vi "BuildExcelTable.vi"(9 "Names":string[](array[string]), 11 "Value":cluster{dbl, "df":dbl, dbl[]}[](array[cluster])) -> (1 "ColHeaders":string[](array[string]), 3 "Breakdown":string[][](table))   [LabVIEW 2022 SP3]
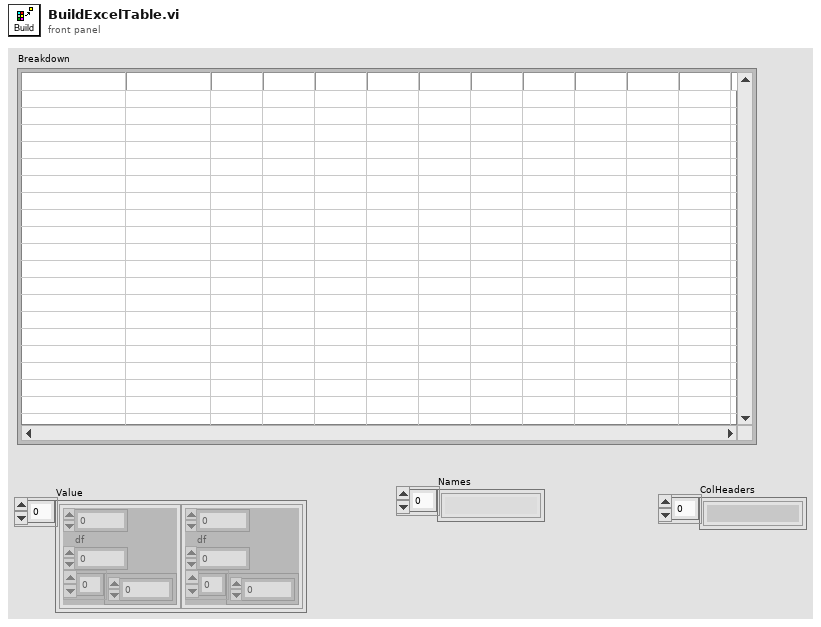
[diagram p1: front panel]
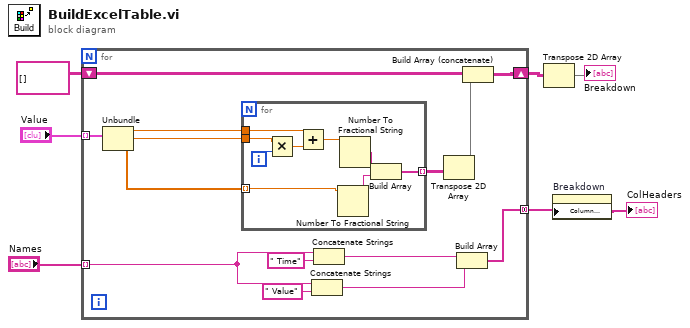
[diagram p0: block diagram]
diagram:
  n1 = for {
    tunnel: "Value" -> [w20] mode=indexing
    shift-right: [w13] -> w2
    shift-left: string[][] [] -> [w12]
    tunnel: [w14] -> w3 mode=concatenating
    tunnel: "Names" -> [w9] mode=indexing
    n2 = Unbundle(w20) -> (w18:dbl, "df"=w19:dbl, w17:dbl[])
    n3 = for {
      tunnel: w19 -> [w28]
      tunnel: w18 -> [w26]
      tunnel: w17 -> [w24] mode=indexing
      tunnel: [w21] -> w16 mode=indexing
      i -> [w29]
      n4 = Multiply(x=w28, y=w29) -> (x*y=w27:dbl)
      n5 = Add(x=w26, y=w27) -> (x+y=w25:dbl)
      n6 = Number To Fractional String(number=w24) -> (F-format string=w23:string)  [unwired: 3 in]
      n7 = Number To Fractional String(number=w25) -> (F-format string=w22:string)  [unwired: 3 in]
      n8 = Build Array(w22, w23) -> (w21:string[])
    }
    n9 = Concatenate Strings(w9, " Value" ("string")) -> (w7:string)
    n10 = Concatenate Strings(w9, " Time" ("string")) -> (w8:string)
    n11 = Transpose 2D Array(2D array=w16) -> (transposed array=w15:string[][])
    n12 = Build Array(w8, w7) -> (w14:string[])
    n13 = Build Array (concatenate)(w12, w15) -> (w13:string[][])
  }
  "ColHeaders" <- w3
  n14 = Transpose 2D Array(2D array=w2) -> (transposed array=→"Breakdown":string[][])
  n15 = property on="Breakdown" class="Tbl (strict)"("Column Headers[]"=w3) -> ()  [unwired: 2 in, 2 out]
